vi "Begin.vi"(11 "Image Size":T1=enum."160x120") -> (0 "error out":errorcluster)   [LabVIEW 2011]
doc: "Called before other user functions, this VI is expected to open initial I/O refnums, load in file data, and do all program initialization. Notice that the <B>error out</B> terminal is simply used for data flow. Wiring it to other structures or subVIs ensures that this VI runs first."
uses:
  <vilib>/Rock Robotics/WPI/Camera/WPI_CameraImageSize.ctl
  <vilib>/Rock Robotics/WPI/Solenoid/WPI_SolenoidChannel.ctl
  <vilib>/Rock Robotics/SystemInterfaces/Typedef/FPGA_TypedefSolenoidModule.ctl
  <vilib>/Rock Robotics/SystemInterfaces/DIO/FPGA_DIOChannel.ctl
  <vilib>/Rock Robotics/SystemInterfaces/Typedef/FPGA_TypedefDigitalModule.ctl
  <vilib>/Rock Robotics/WPI/Solenoid/WPI_SolenoidValue.ctl
  <vilib>/Rock Robotics/WPI/CAN/Jaguar/SubVIs/WPI_CANJaguar_BrakeCoastMode.ctl
  <vilib>/Rock Robotics/WPI/CAN/Jaguar/SubVIs/WPI_CANJaguar_ControlMode.ctl
  <vilib>/Rock Robotics/WPI/Encoder/WPI_EncoderType.ctl
  <vilib>/Rock Robotics/WPI/Joystick/WPI_JoystickDeviceEnum.ctl
  <vilib>/Rock Robotics/SystemInterfaces/DIO/FPGA_DIOPWMChannel.ctl
  <vilib>/Rock Robotics/WPI/Relay/WPI_RelayDirection.ctl
  <vilib>/Rock Robotics/SystemInterfaces/DIO/FPGA_DIORelayChannel.ctl
  <vilib>/Rock Robotics/WPI/Solenoid/WPI_SolenoidOpenDouble.vi
  <vilib>/Rock Robotics/WPI/Counter/WPI_CounterDigitalInputToDigitalSource.vi
  <vilib>/Rock Robotics/WPI/Counter/WPI_CounterOpen Semi Period Mode.vi
  <vilib>/Rock Robotics/WPI/Solenoid/WPI_SolenoidSetEnum.vi
  <vilib>/Rock Robotics/WPI/MotorControl/WPI_MotorControlOpenCANJaguar.vi
  <vilib>/Rock Robotics/WPI/RobotDrive/WPI_RobotDriveOpen4MotorWithJaguar.vi
  <vilib>/Rock Robotics/WPI/Camera/WPI_CameraWhite Balance Values.ctl
  <vilib>/Rock Robotics/WPI/Camera/WPI_CameraExposure Values.ctl
  <vilib>/Rock Robotics/WPI/Camera/WPI_CameraFrameRate.ctl
  <vilib>/Rock Robotics/SystemInterfaces/Typedef/FPGA_TypedefAnalogModuleForGyro.ctl
  <vilib>/Rock Robotics/SystemInterfaces/AI/FPGA_AIGyroChannel.ctl
  <vilib>/Rock Robotics/SystemInterfaces/AI/FPGA_AIChannel.ctl
  <vilib>/Rock Robotics/SystemInterfaces/Typedef/FPGA_TypedefAnalogModule.ctl
  <vilib>/Rock Robotics/WPI/MotorControl/WPI_MotorControlOpen Jaguar.vi
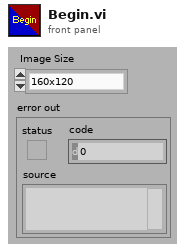
[diagram p1: front panel]
types:
  T1 = typedef "WPI_CameraImageSize.ctl" = enum16{"640x480", "320x240", "160x120"}
  T2 = typedef "FPGA_TypedefDigitalModule.ctl" = enum16{"Digital Module 1", "Digital Module 2"}
  T3 = typedef "FPGA_DIOChannel.ctl" = enum8{"DIO 1", "DIO 2", "DIO 3", "DIO 4", "DIO 5", "DIO 6", "DIO 7", "DIO 8", "DIO 9", "DIO 10", "DIO 11", "DIO 12", "DIO 13", "DIO 14", "Invalid"}
  T4 = typedef "WPI_DigitalInputDevRef.ctl" = cluster{"DevStatus":errorcluster, "DIO Channel":T3, "Digital Module":T2}
  T5 = typedef "WPI_JoystickDeviceEnum.ctl" = enum16{"USB 1", "USB 2", "USB 3", "USB 4", "Kinect 1", "Kinect 2"}
  T6 = typedef "WPI_SolenoidChannel.ctl" = enum8{"Solenoid 1", "Solenoid 2", "Solenoid 3", "Solenoid 4", "Solenoid 5", "Solenoid 6", "Solenoid 7", "Solenoid 8", "Invalid"}
  T7 = typedef "FPGA_TypedefSolenoidModule.ctl" = enum16{"Solenoid Module 1", "Solenoid Module 2"}
  T8 = typedef "FPGA_DIORelayChannel.ctl" = enum8{"Relay 1", "Relay 2", "Relay 3", "Relay 4", "Relay 5", "Relay 6", "Relay 7", "Relay 8", "Invalid"}
  T9 = typedef "WPI_RelayDirection.ctl" = enum16{"Both directions", "Forward only", "Reverse only"}
  T10 = typedef "WPI_EncoderType.ctl" = enum16{"1x", "2x", "4x"}
  T11 = typedef "FPGA_DIOPWMChannel.ctl" = enum8{"PWM 1", "PWM 2", "PWM 3", "PWM 4", "PWM 5", "PWM 6", "PWM 7", "PWM 8", "PWM 9", "PWM 10", "Invalid"}
  T12 = typedef "WPI_JoystickDevRef.ctl" = cluster{"Device":T5}
  T13 = typedef "WPI_RobotDriveDevRef.ctl" = cluster{"DevStatus":errorcluster, "Motors[]":T14[], "Square Inputs":bool, "Max Output":dbl, "Isochronous":bool}
  T14 = typedef "WPI_MotorControlDeviceRef.ctl" = cluster{"DeviceStatus":errorcluster, "Type":enum16{"PWM", "CAN"}, "PWM":cluster{"Digital Module":T2, "PWM Channel":T11, "DeadBand":T15}, "CAN":cluster{"Device Number":u8, "Control Mode":T16, "Semaphore":T17, "Max Vout":dbl}, "Invert":bool, "TransformRef":T18, "InvTransformRef":T18}
  T15 = typedef "WPI_PWMDeadband.ctl" = cluster{"Name":string, "maxPositivePwm":i32, "minPositivePwm":i32, "centerPwm":i32, "maxNegativePwm":i32, "minNegativePwm":i32, "angularRange":u16}
  T16 = typedef "WPI_CANJaguar_ControlMode.ctl" = enum8{"Percent VBus", "Current", "Speed", "Position", "Voltage"}
  T17 = typedef "Semaphore RefNum" = refnum<k1>
  T18 = typedef "WPI_PWMTransform_ConPane.ctl" = refnum<vi>
  T19 = typedef "WPI_SolenoidDevRef.ctl" = cluster{"DevStatus":errorcluster, "Solenoid Module":T7, "Forward Solenoid Channel":T6, "Reverse Solenoid Channel":T6}
  T20 = typedef "WPI_RelayDevRef.ctl" = cluster{"DevStatus":errorcluster, "Relay Channel":T8, "Digital Module":T2, "Relay Direction":T9}
  T21 = typedef "FPGA_CounterEncoderSourceConvertionLVSourceType.ctl" = cluster{"DevStatus":errorcluster, "AnalogTriggerMode?":bool, "DigitalMode":cluster{"Digital Module":T2, "DIO Channel":T22}, "AnalogTriggerMode":cluster{"AnalogTriggerIndex":T23, "OutputType":T24}}
  T22 = typedef "FPGA_DIODigitalSourceChannel.ctl" = enum8{"DIO 1", "DIO 2", "DIO 3", "DIO 4", "DIO 5", "DIO 6", "DIO 7", "DIO 8", "DIO 9", "DIO 10", "DIO 11", "DIO 12", "DIO 13", "DIO 14", "Disabled"}
  T23 = typedef "FPGA_AnalogTriggerIndex.ctl" = enum8{"Trig 0", "Trig 1", "Trig 2", "Trig 3", "Trig 4", "Trig 5", "Trig 6", "Trig 7", "Invalid"}
  T24 = typedef "FPGA_AnalogTriggerOutType.ctl" = enum16{"InWindow", "TriggerState", "Rising", "Falling"}
  T25 = typedef "WPI_EncoderDevRef.ctl" = cluster{"DevStatus":errorcluster, "EncoderIndex":T26, "CounterIndex":T27, "DistancePerCount":dbl, "Decoding Type":T10}
  T26 = typedef "FPGA_EncoderIdx.ctl" = enum8{"Enc 0", "Enc 1", "Enc 2", "Enc 3", "Invalid"}
  T27 = typedef "FPGA_CounterCtrSystemIndex.ctl" = enum8{"Ctr 0", "Ctr 1", "Ctr 2", "Ctr 3", "Ctr 4", "Ctr 5", "Ctr 6", "Ctr 7", "Invalid"}
  T28 = typedef "FPGA_AIChannel.ctl" = enum8{"AI 1", "AI 2", "AI 3", "AI 4", "AI 5", "AI 6", "AI 7", "AI 8", "Invalid"}
  T29 = typedef "FPGA_TypedefAnalogModule.ctl" = enum16{"Analog Module 1", "Analog Module 2"}
  T30 = typedef "FPGA_AIGyroChannel.ctl" = enum8{"AI 1", "AI 2", "Invalid"}
  T31 = typedef "FPGA_TypedefAnalogModuleForGyro.ctl" = enum16{"Analog Module 1"}
  T32 = typedef "WPI_AnalogChannelDevRef.ctl" = cluster{"DevStatus":errorcluster, "Analog Module":T29, "Analog Channel":T28}
  T33 = typedef "WPI_GyroDevRef.ctl" = cluster{"DevStatus":errorcluster, "Analog Module":T29, "Analog Channel":T28, "Offset":dbl, "Gain (VoltsPerDegree/Second)":dbl}
  T34 = cluster{"Channel 1":enum16{"Input (floating)", "Input (pulled high)", "Input (pulled low)", "Output", "PWM"}, "Channel 2":enum16{"Input (floating)", "Input (pulled high)", "Input (pulled low)", "Output", "PWM"}, "Channel 3":enum16{"Input (floating)", "Input (pulled high)", "Input (pulled low)", "Output", "PWM"}, "Channel 4":enum16{"Input (floating)", "Input (pulled high)", "Input (pulled low)", "Output", "PWM"}, "Channel 5":enum16{"Input (floating)", "Input (pulled high)", "Input (pulled low)", "Output"}, "Channel 6":enum16{"Input (floating)", "Input (pulled high)", "Input (pulled low)", "Output"}, "Channel 7":enum16{"Input (floating)", "Input (pulled high)", "Input (pulled low)", "Output"}, "Channel 8":enum16{"Input (floating)", "Input (pulled high)", "Input (pulled low)", "Output"}, "Channel 9":enum16{"Input (floating)", "Input (pulled high)", "Input (pulled low)", "Output"}, "Channel 10":enum16{"Input (floating)", "Input (pulled high)", "Input (pulled low)", "Output"}, "Channel 11":enum16{"Input (floating)", "Input (pulled high)", "Input (pulled low)", "Output"}, "Channel 12":enum16{"Input (floating)", "Input (pulled high)", "Input (pulled low)", "Output"}, "Channel 13":enum16{"Input (floating)", "Input (pulled high)", "Input (pulled low)", "Output"}, "Channel 14":enum16{"Input (floating)", "Input (pulled high)", "Input (pulled low)", "Output"}, "Channel 15":enum16{"Input (floating)", "Input (pulled high)", "Input (pulled low)", "Output", "Analog Comparator"}, "Channel 16":enum16{"Input (floating)", "Input (pulled high)", "Input (pulled low)", "Output", "Analog Comparator"}}
  T35 = cluster{"Period 1(sec)":dbl, "Period 2(sec)":dbl}
  T36 = cluster{"Index Enable 1":bool, "Index Enable 2":bool}
  T37 = typedef "WPI_CameraFrameRate.ctl" = u32
  T38 = typedef "WPI_CameraExposure Values.ctl" = enum16{"Auto", "Flicker-free 50 Hz", "Flicker-free 60 Hz", "Hold current"}
  T39 = typedef "WPI_CameraWhite Balance Values.ctl" = enum16{"Auto", "Fixed indoor", "Fixed outdoor 1", "Fixed outdoor 2", "Fixed fluorescent 1", "Fixed fluorescent 2", "Hold current"}
  T40 = typedef "WPI_CameraDevRef.ctl" = cluster{"Camera Address":string, "CameraStatus":errorcluster, "Acquire Image Notifier":refnum<notifier>}
  T41 = typedef "WPI_SolenoidValue.ctl" = enum16{"Off", "On", "Forward", "Reverse"}
  T42 = typedef "WPI_CounterDevRef.ctl" = cluster{"DevStatus":errorcluster, "CntIndex":T27}
  T43 = typedef "WPI_CANJaguar_BrakeCoastMode.ctl" = enum8{"Jumper", "Brake", "Coast"}
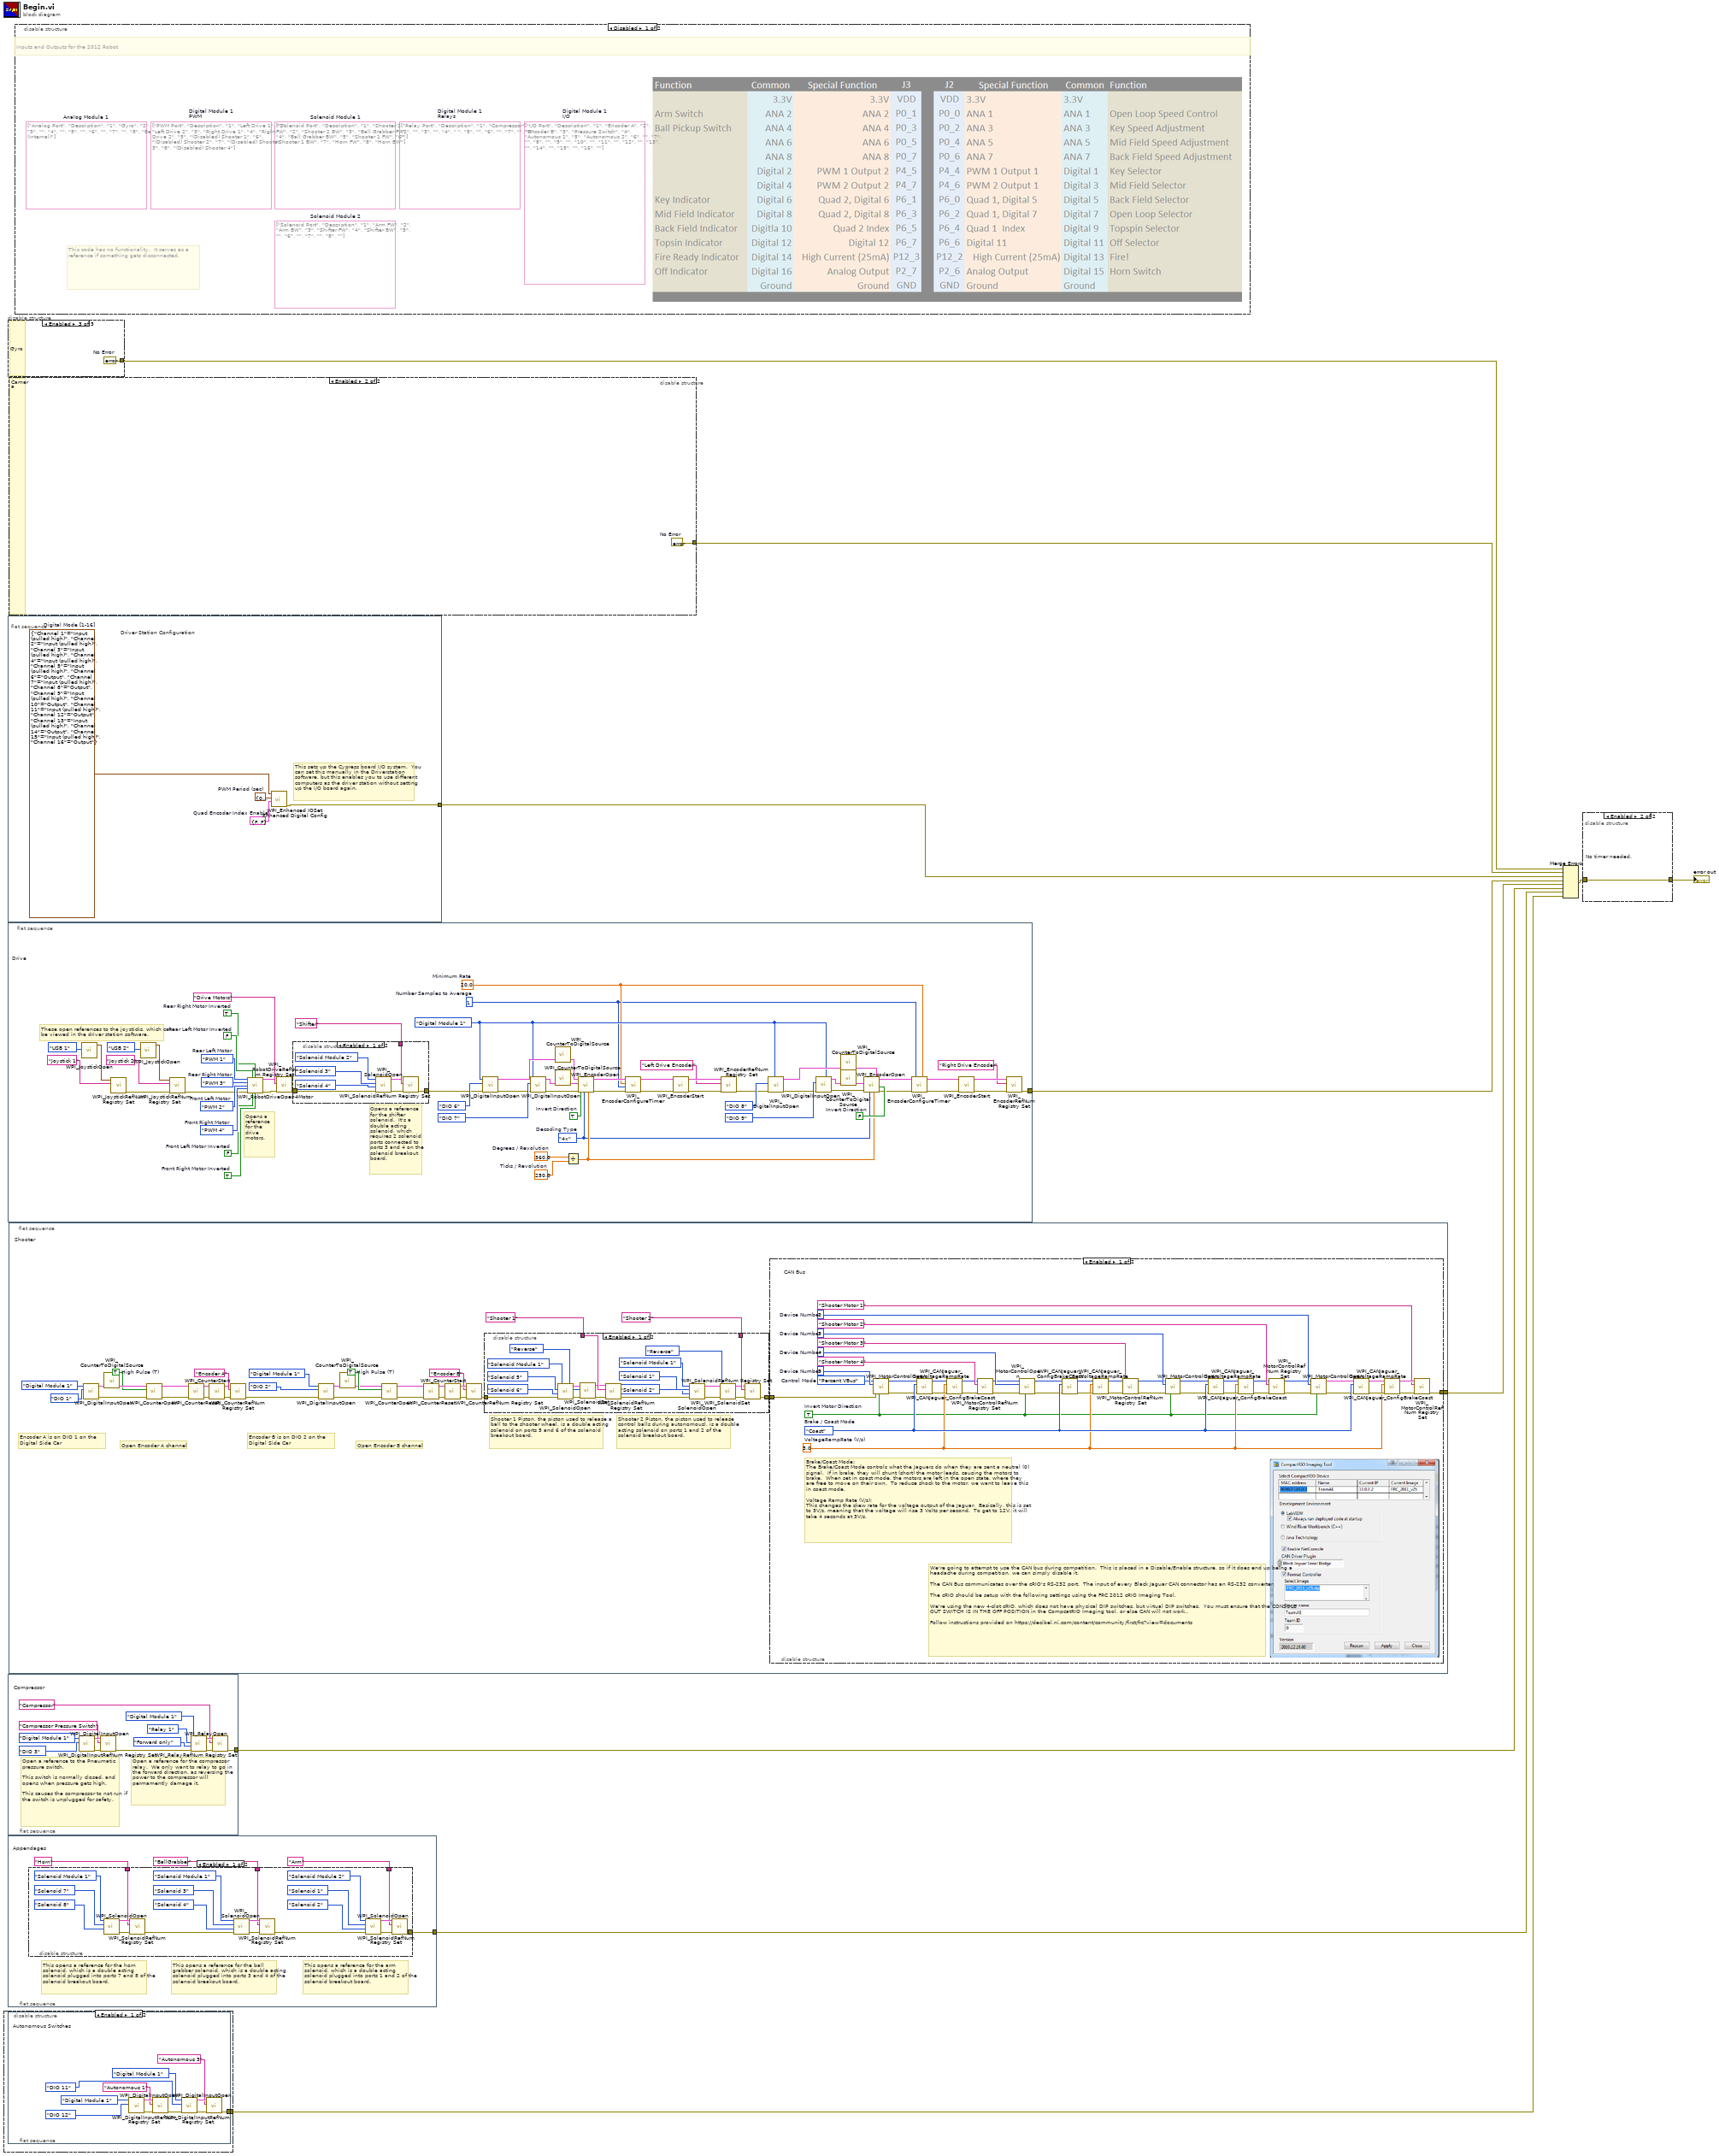
[diagram p0: block diagram]
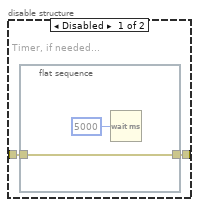
[diagram p4: hidden frame]
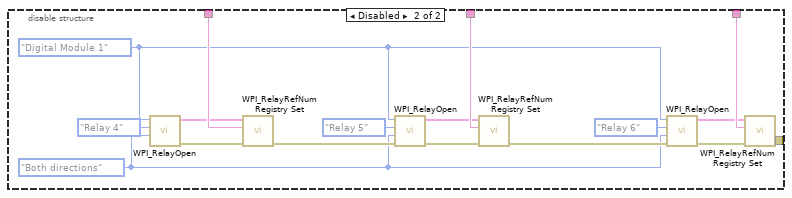
[diagram p5: hidden frame]
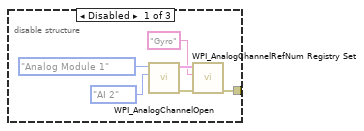
[diagram p6: hidden frame]
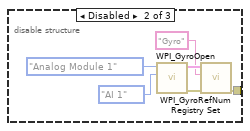
[diagram p7: hidden frame]
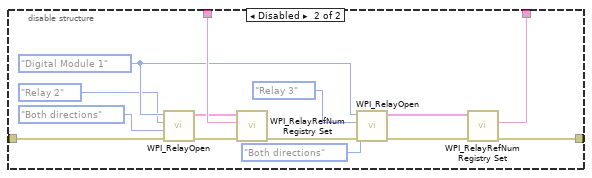
[diagram p8: hidden frame]
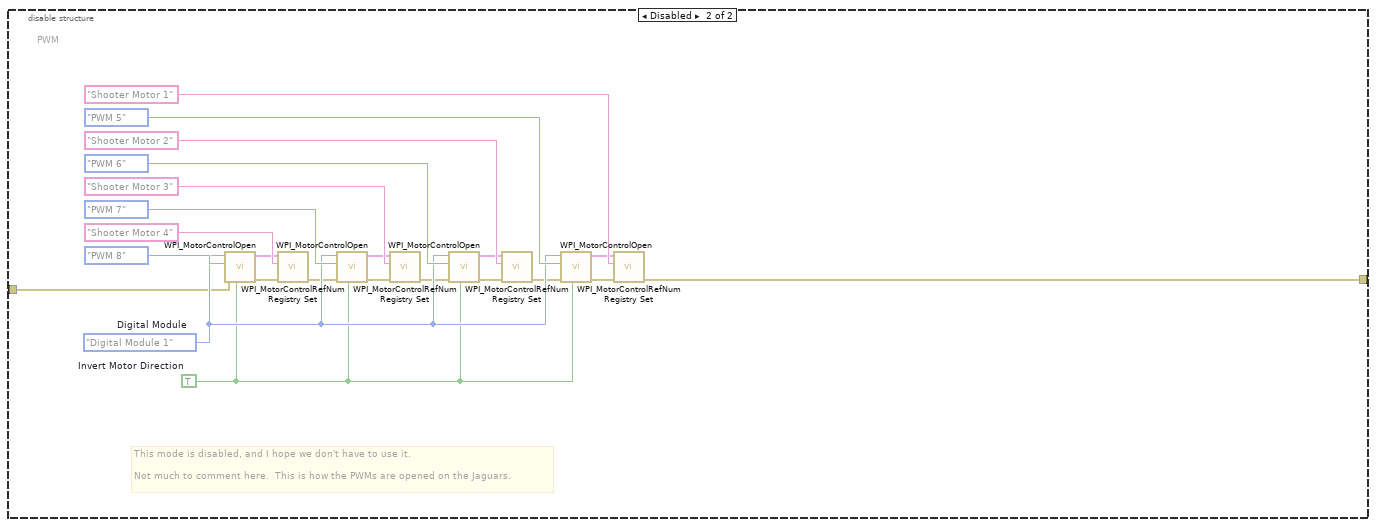
[diagram p9: hidden frame]
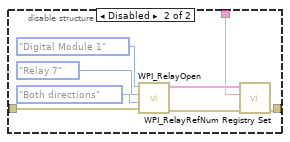
[diagram p10: hidden frame]
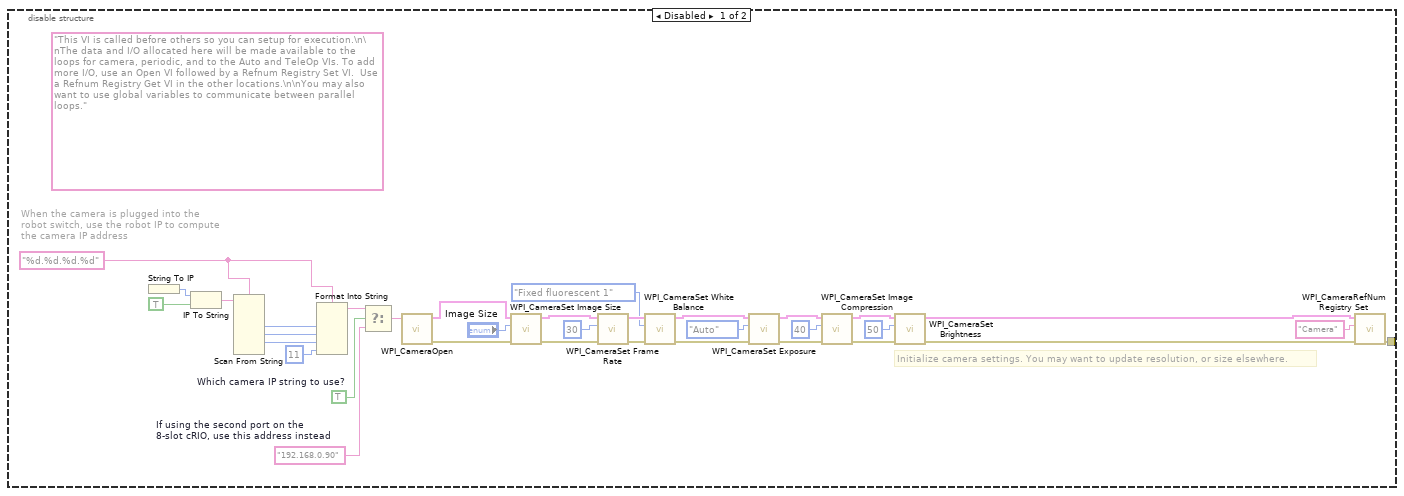
[diagram p11: hidden frame]
diagram:
  n1 = disable-structure shown="Enabled" {
    disable-tunnel: [w11 _] -> w1
    frame Enabled {
      n2 = flat-sequence {
        tunnel: [w12] -> w11
        frame #0 {
          # "Autonomous Switches"
          n3 = call <vilib>:"WPI_DigitalInputOpen.vi"("DIO Channel"=FPGA_DIOChannel."DIO 12", "Digital Module (Module 1)"=FPGA_TypedefDigitalModule."Digital Module 1") -> ("error out"=w19:errorcluster, "DigitalInputDevRef"=w20:T4)  [unwired: 8 in]
          n4 = call <vilib>:"WPI_DigitalInputRefNum Registry Set.vi"("error in (no error)"=w19, "refnum name"="Autonomous 1", "DigitalInputDevRef"=w20) -> ("error out"=w23:errorcluster)  [unwired: 7 in, 1 out]
          n5 = call <vilib>:"WPI_DigitalInputOpen.vi"("error in (no error)"=w23, "DIO Channel"=FPGA_DIOChannel."DIO 11", "Digital Module (Module 1)"=FPGA_TypedefDigitalModule."Digital Module 1") -> ("error out"=w21:errorcluster, "DigitalInputDevRef"=w22:T4)  [unwired: 7 in]
          n6 = call <vilib>:"WPI_DigitalInputRefNum Registry Set.vi"("error in (no error)"=w21, "refnum name"="Autonomous 3", "DigitalInputDevRef"=w22) -> ("error out"=w12:errorcluster)  [unwired: 7 in, 1 out]
        }
      }
    }
    frame Disabled {
    }
  }
  n7 = flat-sequence {
    tunnel: [w35] -> w9
    frame #0 {
      w24 = u8 1  # Number Samples to Average
      w25 = 20.0  # Minimum Rate
      w64 = 250.0  # Ticks / Revolution
      w52 = TRUE  # Invert Direction
      w61 = FALSE  # Invert Direction
      w27 = WPI_EncoderType."4x"  # Decoding Type
      w26 = FPGA_TypedefDigitalModule."Digital Module 1" ("DIO Module")
      w65 = 360.0  # Degrees / Revolution
      w73 = TRUE  # Front Right Motor Inverted
      w74 = FALSE  # Front Left Motor Inverted
      w75 = TRUE  # Rear Right Motor Inverted
      w76 = FALSE  # Rear Left Motor Inverted
      w77 = FPGA_DIOPWMChannel."PWM 4"  # Front Right Motor
      w78 = FPGA_DIOPWMChannel."PWM 2"  # Front Left Motor
      w79 = FPGA_DIOPWMChannel."PWM 3"  # Rear Right Motor
      w80 = FPGA_DIOPWMChannel."PWM 1"  # Rear Left Motor
      # "Opens a reference for the shifter solenoid.  It's a double acting solenoid, which requires 2 solenoid ports connected to ports 3 and 4 on the solenoid breakout board."
      # "Opens a reference for the drive motors."
      # "These open references to the joysticks, which can be viewed in the driver station software."
      # "Drive"
      n8 = call <vilib>:"WPI_JoystickOpen.vi"("JoystickDevice"=WPI_JoystickDeviceEnum."USB 1") -> ("JoystickDevRef"=w85:T12)  [unwired: 10 out]
      n9 = call <vilib>:"WPI_JoystickRefNum Registry Set.vi"("refnum name"="Joystick 1", "JoystickDevRef"=w85) -> ("error out"=w66:errorcluster)  [unwired: 1 in, 8 out]
      n10 = call <vilib>:"WPI_JoystickOpen.vi"("JoystickDevice"=WPI_JoystickDeviceEnum."USB 2") -> ("JoystickDevRef"=w71:T12)  [unwired: 10 out]
      n11 = call <vilib>:"WPI_JoystickRefNum Registry Set.vi"("error in (no error)"=w66, "refnum name"="Joystick 2", "JoystickDevRef"=w71) -> ("error out"=w67:errorcluster)  [unwired: 8 out]
      n12 = call-poly <vilib>:"WPI_RobotDriveOpen4Motor.vi"("Rear Left Motor"=w80, "Rear Left Motor Inverted"=w76, "Rear Right Motor Inverted"=w75, "Rear Right Motor"=w79, "Front Left Motor"=w78, "Front Right Motor"=w77, "error in (no error)"=w67, "Front Left Motor Inverted"=w74, "Front Right Motor Inverted"=w73) -> ("RobotDriveDevRef"=w82:T13, "error out"=w81:errorcluster)  [unwired: 5 in]
      n13 = call <vilib>:"WPI_RobotDriveRefNum Registry Set.vi"("error in (no error)"=w81, "refnum name"="Drive Motors", "RobotDriveDevRef"=w82) -> ("error out"=w68:errorcluster)  [unwired: 8 out]
      n14 = disable-structure shown="Enabled" {
        disable-tunnel: "Shifter" ("refnum name") -> [w93 w98]
        disable-tunnel: w68 -> [w88 w102]
        disable-tunnel: [w87 w100] -> w34
        frame Enabled {
          n15 = call-poly <vilib>:"WPI_SolenoidOpen.vi"("error in (no error)"=w88, "Reverse Solenoid Channel"=WPI_SolenoidChannel."Solenoid 4", "Forward Solenoid Channel"=WPI_SolenoidChannel."Solenoid 3", "Solenoid Module (Module 1)"=FPGA_TypedefSolenoidModule."Solenoid Module 2") -> ("error out"=w91:errorcluster, "SolenoidDevRef"=w90:T19)  [unwired: 6 in]
          n16 = call <vilib>:"WPI_SolenoidRefNum Registry Set.vi"("error in (no error)"=w91, "refnum name"=w93, "SolenoidDevRef"=w90) -> ("error out"=w87:errorcluster)  [unwired: 7 in, 1 out]
        }
        frame Disabled {
          n17 = call <vilib>:"WPI_RelayOpen.vi"("error in (no error)"=w102, "Relay Direction"=WPI_RelayDirection."Both directions", "Relay Channel"=FPGA_DIORelayChannel."Relay 7", "Digital Module (Module 1)"=FPGA_TypedefDigitalModule."Digital Module 1") -> ("error out"=w101:errorcluster, "RelayDevRef"=w99:T20)  [unwired: 6 in]
          n18 = call <vilib>:"WPI_RelayRefNum Registry Set.vi"("error in (no error)"=w101, "refnum name"=w98, "RelayDevRef"=w99) -> ("error out"=w100:errorcluster)  [unwired: 7 in, 1 out]
        }
      }
      n19 = call <vilib>:"WPI_DigitalInputOpen.vi"("error in (no error)"=w34, "DIO Channel"=FPGA_DIOChannel."DIO 6", "Digital Module (Module 1)"=w26) -> ("error out"=w33:errorcluster, "DigitalInputDevRef"=w50:T4)  [unwired: 7 out]
      n20 = call <vilib>:"WPI_DigitalInputOpen.vi"("error in (no error)"=w33, "DIO Channel"=FPGA_DIOChannel."DIO 7", "Digital Module (Module 1)"=w26) -> ("error out"=w32:errorcluster, "DigitalInputDevRef"=w49:T4)  [unwired: 7 out]
      n21 = call-poly <vilib>:"WPI_CounterToDigitalSource.vi"("DigitalInputDevRef"=w50) -> ("Digital Source"=w51:T21)  [unwired: 6 out]
      n22 = call-poly <vilib>:"WPI_CounterToDigitalSource.vi"("DigitalInputDevRef"=w49) -> ("Digital Source"=w48:T21)  [unwired: 6 out]
      n23 = Divide(x=w65, y=w64) -> (x/y=w28:dbl)
      n24 = call <vilib>:"WPI_EncoderOpen.vi"("DistancePerCount"=w28, "Decoding Type"=w27, "error in (no error)"=w32, "Invert Direction (False)"=w52, "BSource"=w48, "ASource"=w51) -> ("error out"=w47:errorcluster, "EncoderDevRef"=w46:T25)  [unwired: 2 in, 2 out]
      n25 = call <vilib>:"WPI_EncoderConfigureTimer.vi"("error in (no error)"=w47, "Number Samples to Average"=w24, "Minimum Rate"=w25, "EncoderDevRef"=w46) -> ("error out"=w42:errorcluster, "EncoderDevRef"=w45:T25)  [unwired: 6 out]
      n26 = call <vilib>:"WPI_EncoderStart.vi"("error in (no error)"=w42, "EncoderDevRef"=w45) -> ("error out"=w41:errorcluster, "EncoderDevRef"=w40:T25)  [unwired: 8 out]
      n27 = call <vilib>:"WPI_EncoderRefNum Registry Set.vi"("error in (no error)"=w41, "refnum name"="Left Drive Encoder", "EncoderDevRef"=w40) -> ("error out"=w31:errorcluster)  [unwired: 7 in, 1 out]
      n28 = call <vilib>:"WPI_DigitalInputOpen.vi"("error in (no error)"=w31, "DIO Channel"=FPGA_DIOChannel."DIO 8" ("Encoder A Channel"), "Digital Module (Module 1)"=w26) -> ("error out"=w30:errorcluster, "DigitalInputDevRef"=w58:T4)  [unwired: 7 out]
      n29 = call <vilib>:"WPI_DigitalInputOpen.vi"("error in (no error)"=w30, "DIO Channel"=FPGA_DIOChannel."DIO 9" ("Encoder B Channel"), "Digital Module (Module 1)"=w26) -> ("error out"=w29:errorcluster, "DigitalInputDevRef"=w59:T4)  [unwired: 7 out]
      n30 = call-poly <vilib>:"WPI_CounterToDigitalSource.vi"("DigitalInputDevRef"=w58) -> ("Digital Source"=w57:T21)  [unwired: 6 out]
      n31 = call-poly <vilib>:"WPI_CounterToDigitalSource.vi"("DigitalInputDevRef"=w59) -> ("Digital Source"=w60:T21)  [unwired: 6 out]
      n32 = call <vilib>:"WPI_EncoderOpen.vi"("DistancePerCount"=w28, "Decoding Type"=w27, "error in (no error)"=w29, "Invert Direction (False)"=w61, "BSource"=w60, "ASource"=w57) -> ("error out"=w44:errorcluster, "EncoderDevRef"=w55:T25)  [unwired: 2 in, 2 out]
      n33 = call <vilib>:"WPI_EncoderConfigureTimer.vi"("error in (no error)"=w44, "Number Samples to Average"=w24, "Minimum Rate"=w25, "EncoderDevRef"=w55) -> ("error out"=w43:errorcluster, "EncoderDevRef"=w56:T25)  [unwired: 6 out]
      n34 = call <vilib>:"WPI_EncoderStart.vi"("error in (no error)"=w43, "EncoderDevRef"=w56) -> ("error out"=w39:errorcluster, "EncoderDevRef"=w38:T25)  [unwired: 8 out]
      n35 = call <vilib>:"WPI_EncoderRefNum Registry Set.vi"("error in (no error)"=w39, "refnum name"="Right Drive Encoder", "EncoderDevRef"=w38) -> ("error out"=w35:errorcluster)  [unwired: 7 in, 1 out]
    }
  }
  n36 = disable-structure shown="Enabled" {
    disable-tunnel: [w103 w109 w115] -> w2
    frame Disabled {
      n37 = call <vilib>:"WPI_AnalogChannelOpen.vi"("Analog Channel"=FPGA_AIChannel."AI 2", "Analog Module (Module 1)"=FPGA_TypedefAnalogModule."Analog Module 1") -> ("error out"=w104:errorcluster, "AIDeviceRef"=w108:T32)  [unwired: 8 in]
      n38 = call <vilib>:"WPI_AnalogChannelRefNum Registry Set.vi"("error in (no error)"=w104, "refnum name"="Gyro", "AIDeviceRef"=w108) -> ("error out"=w103:errorcluster)  [unwired: 7 in, 1 out]
    }
    frame Disabled {
      n39 = call <vilib>:"WPI_GyroOpen.vi"("Analog Channel"=FPGA_AIGyroChannel."AI 1", "Analog Module (Module 1)"=FPGA_TypedefAnalogModuleForGyro."Analog Module 1") -> ("error out"=w114:errorcluster, "GyroDevRef"=w113:T33)  [unwired: 7 in, 1 out]
      n40 = call <vilib>:"WPI_GyroRefNum Registry Set.vi"("error in (no error)"=w114, "refnum name"="Gyro", "GyroDevRef"=w113) -> ("error out"=w109:errorcluster)  [unwired: 7 in, 1 out]
    }
    frame Enabled {
      w115 = errorcluster {"status"=FALSE, "code"=0, "source"=""}  # No Error
      # "Gyro"
    }
  }
  n41 = flat-sequence {
    tunnel: [w116] -> w10
    frame #0 {
      w117 = T34 {"Channel 1"=enum."Input (pulled high)", "Channel 2"=enum."Input (pulled high)", "Channel 3"=enum."Input (pulled high)", "Channel 4"=enum."Input (pulled high)", "Channel 5"=enum."Input (pulled high)", "Channel 6"=enum."Output", "Channel 7"=enum."Input (pulled high)", "Channel 8"=enum."Output", "Channel 9"=enum."Input (pulled high)", "Channel 10"=enum."Output", "Channel 11"=enum."Input (pulled high)", "Channel 12"=enum."Output", "Channel 13"=enum."Input (pulled high)", "Channel 14"=enum."Output", "Channel 15"=enum."Input (pulled high)", "Channel 16"=enum."Output"}  # Digital Mode [1-16]
      w118 = T35 {"Period 1(sec)"=0.0, "Period 2(sec)"=0.0}  # PWM Period (sec)
      w119 = T36 {"Index Enable 1"=FALSE, "Index Enable 2"=FALSE}  # Quad Encoder Index Enable
      # "This sets up the Cypress board I/O system.  You can set this manually in the Driverstation software, but this enables you to use different computers as the driver station without setting up the I/O board again."
      # "Driver Station Configuration"
      n42 = call <vilib>:"WPI_Enhanced IOSet Enhanced Digital Config.vi"("Quad Encoder Index Enable"=w119, "PWM Period (sec)"=w118, "Digital Mode [1-16]"=w117) -> ("error out"=w116:errorcluster)  [unwired: 8 in]
    }
  }
  n43 = flat-sequence {
    tunnel: [w120] -> w7
    frame #0 {
      # "Open a reference for the compressor relay.  We only want to relay to go in the forward direction, as reversing the power to the compressor will permamently damage it."
      # "Open a reference to the Pneumatic pressure switch.\n\nThis switch is normally closed, and opens when pressure gets high.\n\nThis causes the compressor to not run if the switch is unplugged for safety."
      # "Compressor"
      n44 = call <vilib>:"WPI_DigitalInputOpen.vi"("DIO Channel"=FPGA_DIOChannel."DIO 3", "Digital Module (Module 1)"=FPGA_TypedefDigitalModule."Digital Module 1") -> ("error out"=w125:errorcluster, "DigitalInputDevRef"=w126:T4)  [unwired: 8 in]
      n45 = call <vilib>:"WPI_DigitalInputRefNum Registry Set.vi"("error in (no error)"=w125, "refnum name"="Compressor Pressure Switch", "DigitalInputDevRef"=w126) -> ("error out"=w121:errorcluster)  [unwired: 7 in, 1 out]
      n46 = call <vilib>:"WPI_RelayOpen.vi"("error in (no error)"=w121, "Relay Direction"=WPI_RelayDirection."Forward only", "Relay Channel"=FPGA_DIORelayChannel."Relay 1", "Digital Module (Module 1)"=FPGA_TypedefDigitalModule."Digital Module 1") -> ("error out"=w131:errorcluster, "RelayDevRef"=w132:T20)  [unwired: 6 in]
      n47 = call <vilib>:"WPI_RelayRefNum Registry Set.vi"("error in (no error)"=w131, "refnum name"="Compressor", "RelayDevRef"=w132) -> ("error out"=w120:errorcluster)  [unwired: 7 in, 1 out]
    }
  }
  n48 = flat-sequence {
    tunnel: [w133] -> w6
    frame #0 {
      # "This opens a reference for the arm solenoid, which is a double acting solenoid plugged into ports 1 and 2 of the solenoid breakout board."
      # "This opens a reference for the ball grabber solenoid, which is a double acting solenoid plugged into ports 3 and 4 of the solenoid breakout board."
      # "This opens a reference for the horn solenoid, which is a double acting solenoid plugged into ports 7 and 8 of the solenoid breakout board."
      # "Appendages"
      n49 = disable-structure shown="Enabled" {
        disable-tunnel: "BallGrabber" ("refnum name") -> [w148 w167]
        disable-tunnel: "Horn" ("refnum name") -> [w147 w168]
        disable-tunnel: "Arm" ("refnum name") -> [w146 w166]
        disable-tunnel: [w137 w174] -> w133
        frame Enabled {
          n50 = call-poly <vilib>:"WPI_SolenoidOpen.vi"("Reverse Solenoid Channel"=WPI_SolenoidChannel."Solenoid 8", "Forward Solenoid Channel"=WPI_SolenoidChannel."Solenoid 7", "Solenoid Module (Module 1)"=FPGA_TypedefSolenoidModule."Solenoid Module 1") -> ("error out"=w154:errorcluster, "SolenoidDevRef"=w155:T19)  [unwired: 7 in]
          n51 = call <vilib>:"WPI_SolenoidRefNum Registry Set.vi"("error in (no error)"=w154, "refnum name"=w147, "SolenoidDevRef"=w155) -> ("error out"=w139:errorcluster)  [unwired: 7 in, 1 out]
          n52 = call-poly <vilib>:"WPI_SolenoidOpen.vi"("error in (no error)"=w139, "Reverse Solenoid Channel"=WPI_SolenoidChannel."Solenoid 4", "Forward Solenoid Channel"=WPI_SolenoidChannel."Solenoid 3", "Solenoid Module (Module 1)"=FPGA_TypedefSolenoidModule."Solenoid Module 1") -> ("error out"=w157:errorcluster, "SolenoidDevRef"=w156:T19)  [unwired: 6 in]
          n53 = call <vilib>:"WPI_SolenoidRefNum Registry Set.vi"("error in (no error)"=w157, "refnum name"=w148, "SolenoidDevRef"=w156) -> ("error out"=w138:errorcluster)  [unwired: 7 in, 1 out]
          n54 = call-poly <vilib>:"WPI_SolenoidOpen.vi"("error in (no error)"=w138, "Reverse Solenoid Channel"=WPI_SolenoidChannel."Solenoid 2", "Forward Solenoid Channel"=WPI_SolenoidChannel."Solenoid 1", "Solenoid Module (Module 1)"=FPGA_TypedefSolenoidModule."Solenoid Module 2") -> ("error out"=w152:errorcluster, "SolenoidDevRef"=w153:T19)  [unwired: 6 in]
          n55 = call <vilib>:"WPI_SolenoidRefNum Registry Set.vi"("error in (no error)"=w152, "refnum name"=w146, "SolenoidDevRef"=w153) -> ("error out"=w137:errorcluster)  [unwired: 7 in, 1 out]
        }
        frame Disabled {
          w161 = WPI_RelayDirection."Both directions" ("Relay Direction")
          w162 = FPGA_TypedefDigitalModule."Digital Module 1" ("Digital Module (Module 1)")
          n56 = call <vilib>:"WPI_RelayOpen.vi"("Relay Direction"=w161, "Relay Channel"=FPGA_DIORelayChannel."Relay 4", "Digital Module (Module 1)"=w162) -> ("error out"=w169:errorcluster, "RelayDevRef"=w163:T20)  [unwired: 7 in]
          n57 = call <vilib>:"WPI_RelayRefNum Registry Set.vi"("error in (no error)"=w169, "refnum name"=w168, "RelayDevRef"=w163) -> ("error out"=w170:errorcluster)  [unwired: 7 in, 1 out]
          n58 = call <vilib>:"WPI_RelayOpen.vi"("error in (no error)"=w170, "Relay Direction"=w161, "Relay Channel"=FPGA_DIORelayChannel."Relay 5", "Digital Module (Module 1)"=w162) -> ("error out"=w171:errorcluster, "RelayDevRef"=w164:T20)  [unwired: 6 in]
          n59 = call <vilib>:"WPI_RelayRefNum Registry Set.vi"("error in (no error)"=w171, "refnum name"=w167, "RelayDevRef"=w164) -> ("error out"=w172:errorcluster)  [unwired: 7 in, 1 out]
          n60 = call <vilib>:"WPI_RelayOpen.vi"("error in (no error)"=w172, "Relay Direction"=w161, "Relay Channel"=FPGA_DIORelayChannel."Relay 6", "Digital Module (Module 1)"=w162) -> ("error out"=w173:errorcluster, "RelayDevRef"=w165:T20)  [unwired: 6 in]
          n61 = call <vilib>:"WPI_RelayRefNum Registry Set.vi"("error in (no error)"=w173, "refnum name"=w166, "RelayDevRef"=w165) -> ("error out"=w174:errorcluster)  [unwired: 7 in, 1 out]
        }
      }
    }
  }
  n62 = disable-structure shown="Enabled" {
    disable-tunnel: [w175 w209] -> w3
    frame Disabled {
      w176 = TRUE  # Which camera IP string to use?
      w180 = "%d.%d.%d.%d" ("format string")
      (unwired) "This VI is called before others so you can setup for execution.\n\nThe data and I/O allocated here will be made available to the loops for camera, periodic, and to the Auto and TeleOp VIs. To add more I/O, use an Open VI followed by a Refnum Registry Set VI.  Use a Refnum Registry Get VI in the other locations.\n\nYou may also want to use global variables to communicate between parallel loops."
      w177 = "192.168.0.90"  # If using the second port on the 8-slot cRIO, use this address instead
      # "When the camera is plugged into the\nrobot switch, use the robot IP to compute\nthe camera IP address"
      # "Initialize camera settings. You may want to update resolution, or size elsewhere."
      n63 = String To IP() -> (0:w187:u32)  [unwired: 1 in]
      n64 = IP To String(1:TRUE ("dot notation? (F)"), 2:w187) -> (0:w185:string)
      n65 = Scan From String(format string=w180, input string=w185) -> (output 1=w184:i32, output 2=w183:i32, output 3=w182:i32)  [unwired: 7 in, 3 out]
      n66 = Format Into String(format string=w180, w184, w183, w182, 11 ("Compression")) -> (resulting string=w178:string)  [unwired: 2 in, 1 out]
      n67 = Select(t=w178, s=w176, f=w177) -> (s? t:f=w179:string)
      n68 = call <vilib>:"WPI_CameraOpen.vi"("Camera Address"=w179) -> ("error out"=w199:errorcluster, "CameraDevRef"=w200:T40)  [unwired: 1 in, 8 out]
      n69 = call <vilib>:"WPI_CameraSet Image Size.vi"("error in (no error)"=w199, "Image Size"="Image Size", "CameraDevRef"=w200) -> ("error out"=w198:errorcluster, "CameraDevRef Out"=w201:T40)  [unwired: 7 out]
      n70 = call <vilib>:"WPI_CameraSet Frame Rate.vi"("error in (no error)"=w198, "Frame Rate (fps)"=T37 30, "CameraDevRef"=w201) -> ("error out"=w197:errorcluster, "CameraDevRef Out"=w203:T40)  [unwired: 7 out]
      n71 = call <vilib>:"WPI_CameraSet White Balance.vi"("error in (no error)"=w197, "White Balance"=WPI_CameraWhite_Balance_Values."Fixed fluorescent 1", "CameraDevRef"=w203) -> ("error out"=w196:errorcluster, "CameraDevRef Out"=w202:T40)  [unwired: 7 out]
      n72 = call <vilib>:"WPI_CameraSet Exposure.vi"("error in (no error)"=w196, "Exposure"=WPI_CameraExposure_Values."Auto", "CameraDevRef"=w202) -> ("error out"=w195:errorcluster, "CameraDevRef Out"=w205:T40)  [unwired: 7 out]
      n73 = call <vilib>:"WPI_CameraSet Image Compression.vi"("error in (no error)"=w195, "Compression"=40, "CameraDevRef"=w205) -> ("error out"=w194:errorcluster, "CameraDevRef Out"=w204:T40)  [unwired: 7 out]
      n74 = call <vilib>:"WPI_CameraSet Brightness.vi"("error in (no error)"=w194, "Brightness"=50, "CameraDevRef"=w204) -> ("error out"=w192:errorcluster, "CameraDevRef Out"=w193:T40)  [unwired: 7 out]
      n75 = call <vilib>:"WPI_CameraRefNum Registry Set.vi"("error in (no error)"=w192, "refnum name"="Camera", "CameraDevRef"=w193) -> ("error out"=w175:errorcluster)  [unwired: 8 out]
    }
    frame Enabled {
      w209 = errorcluster {"status"=FALSE, "code"=0, "source"=""}  # No Error
      # "Camera"
    }
  }
  n76 = flat-sequence {
    tunnel: [w212] -> w8
    frame #0 {
      w226 = TRUE  # High Pulse (T)
      w231 = TRUE  # High Pulse (T)
      # "Shooter 2 Piston, the piston used to release control balls during autonomousl, is a double acting solenoid on ports 1 and 2 of the solenoid breakout board."
      # "Shooter 1 Piston, the piston used to release a ball to the shooter wheel, is a double acting solenoid on ports 5 and 6 of the solenoid breakout board."
      # "Encoder A is on DIO 1 on the Digital Side Car"
      # "Encoder B is on DIO 2 on the Digital Side Car"
      # "Open Encoder B channel"
      # "Open Encoder A channel"
      # "Shooter"
      n77 = call <vilib>:"WPI_DigitalInputOpen.vi"("DIO Channel"=FPGA_DIOChannel."DIO 1", "Digital Module (Module 1)"=FPGA_TypedefDigitalModule."Digital Module 1") -> ("error out"=w232:errorcluster, "DigitalInputDevRef"=w233:T4)  [unwired: 8 in]
      n78 = call-poly <vilib>:"WPI_CounterToDigitalSource.vi"("DigitalInputDevRef"=w233) -> ("Digital Source"=w241:T21)  [unwired: 6 in]
      n79 = call-poly <vilib>:"WPI_CounterOpen.vi"("error in (no error)"=w232, "High Pulse (T)"=w231, "Source"=w241) -> ("error out"=w237:errorcluster, "CounterDevRef"=w238:T42)  [unwired: 7 in]
      n80 = call <vilib>:"WPI_CounterReset.vi"("error in (no error)"=w237, "CounterDevRef in"=w238) -> ("error out"=w236:errorcluster, "CounterDevRef out"=w239:T42)  [unwired: 8 in]
      n81 = call <vilib>:"WPI_CounterStart.vi"("error in (no error)"=w236, "CounterDevRef in"=w239) -> ("error out"=w234:errorcluster, "CounterDevRef out"=w235:T42)  [unwired: 8 in]
      n82 = call <vilib>:"WPI_CounterRefNum Registry Set.vi"("error in (no error)"=w234, "refnum name"="Encoder A", "CounterDevRef"=w235) -> ("error out"=w215:errorcluster)  [unwired: 7 in, 1 out]
      n83 = call <vilib>:"WPI_DigitalInputOpen.vi"("error in (no error)"=w215, "DIO Channel"=FPGA_DIOChannel."DIO 2", "Digital Module (Module 1)"=FPGA_TypedefDigitalModule."Digital Module 1") -> ("error out"=w225:errorcluster, "DigitalInputDevRef"=w224:T4)  [unwired: 7 in]
      n84 = call-poly <vilib>:"WPI_CounterToDigitalSource.vi"("DigitalInputDevRef"=w224) -> ("Digital Source"=w216:T21)  [unwired: 6 in]
      n85 = call-poly <vilib>:"WPI_CounterOpen.vi"("error in (no error)"=w225, "High Pulse (T)"=w226, "Source"=w216) -> ("error out"=w220:errorcluster, "CounterDevRef"=w219:T42)  [unwired: 7 in]
      n86 = call <vilib>:"WPI_CounterReset.vi"("error in (no error)"=w220, "CounterDevRef in"=w219) -> ("error out"=w221:errorcluster, "CounterDevRef out"=w218:T42)  [unwired: 8 in]
      n87 = call <vilib>:"WPI_CounterStart.vi"("error in (no error)"=w221, "CounterDevRef in"=w218) -> ("error out"=w223:errorcluster, "CounterDevRef out"=w222:T42)  [unwired: 8 in]
      n88 = call <vilib>:"WPI_CounterRefNum Registry Set.vi"("error in (no error)"=w223, "refnum name"="Encoder B", "CounterDevRef"=w222) -> ("error out"=w214:errorcluster)  [unwired: 7 in, 1 out]
      n89 = disable-structure shown="Enabled" {
        disable-tunnel: w214 -> [w256 w274]
        disable-tunnel: [w254 w270] -> w213
        disable-tunnel: "Shooter 2" ("refnum name") -> [w253 w275]
        disable-tunnel: "Shooter 1" ("refnum name") -> [w252 w276]
        frame Enabled {
          n90 = call-poly <vilib>:"WPI_SolenoidOpen.vi"("error in (no error)"=w256, "Reverse Solenoid Channel"=WPI_SolenoidChannel."Solenoid 6", "Forward Solenoid Channel"=WPI_SolenoidChannel."Solenoid 5", "Solenoid Module (Module 1)"=FPGA_TypedefSolenoidModule."Solenoid Module 1") -> ("error out"=w249:errorcluster, "SolenoidDevRef"=w250:T19)  [unwired: 6 in]
          n91 = call-poly <vilib>:"WPI_SolenoidSet.vi"("error in (no error)"=w249, "Value"=WPI_SolenoidValue."Reverse", "SolenoidDevRef"=w250) -> ("error out"=w247:errorcluster, "SolenoidDevRef"=w248:T19)  [unwired: 7 in]
          n92 = call <vilib>:"WPI_SolenoidRefNum Registry Set.vi"("error in (no error)"=w247, "refnum name"=w252, "SolenoidDevRef"=w248) -> ("error out"=w255:errorcluster)  [unwired: 7 in, 1 out]
          n93 = call-poly <vilib>:"WPI_SolenoidOpen.vi"("error in (no error)"=w255, "Reverse Solenoid Channel"=WPI_SolenoidChannel."Solenoid 2", "Forward Solenoid Channel"=WPI_SolenoidChannel."Solenoid 1", "Solenoid Module (Module 1)"=FPGA_TypedefSolenoidModule."Solenoid Module 1") -> ("error out"=w242:errorcluster, "SolenoidDevRef"=w245:T19)  [unwired: 6 in]
          n94 = call-poly <vilib>:"WPI_SolenoidSet.vi"("error in (no error)"=w242, "Value"=WPI_SolenoidValue."Reverse", "SolenoidDevRef"=w245) -> ("error out"=w243:errorcluster, "SolenoidDevRef"=w244:T19)  [unwired: 7 in]
          n95 = call <vilib>:"WPI_SolenoidRefNum Registry Set.vi"("error in (no error)"=w243, "refnum name"=w253, "SolenoidDevRef"=w244) -> ("error out"=w254:errorcluster)  [unwired: 7 in, 1 out]
        }
        frame Disabled {
          w267 = FPGA_TypedefDigitalModule."Digital Module 1" ("Digital Module (Module 1)")
          n96 = call <vilib>:"WPI_RelayOpen.vi"("error in (no error)"=w274, "Relay Direction"=WPI_RelayDirection."Both directions", "Relay Channel"=FPGA_DIORelayChannel."Relay 2", "Digital Module (Module 1)"=w267) -> ("error out"=w273:errorcluster, "RelayDevRef"=w268:T20)  [unwired: 6 in]
          n97 = call <vilib>:"WPI_RelayRefNum Registry Set.vi"("error in (no error)"=w273, "refnum name"=w276, "RelayDevRef"=w268) -> ("error out"=w272:errorcluster)  [unwired: 7 in, 1 out]
          n98 = call <vilib>:"WPI_RelayOpen.vi"("error in (no error)"=w272, "Relay Direction"=WPI_RelayDirection."Both directions", "Relay Channel"=FPGA_DIORelayChannel."Relay 3", "Digital Module (Module 1)"=w267) -> ("error out"=w271:errorcluster, "RelayDevRef"=w269:T20)  [unwired: 6 in]
          n99 = call <vilib>:"WPI_RelayRefNum Registry Set.vi"("error in (no error)"=w271, "refnum name"=w275, "RelayDevRef"=w269) -> ("error out"=w270:errorcluster)  [unwired: 7 in, 1 out]
        }
      }
      n100 = disable-structure shown="Enabled" {
        disable-tunnel: w213 -> [w278 w323]
        disable-tunnel: [w277 w319] -> w212
        frame Enabled {
          w279 = TRUE  # Invert Motor Direction
          w300 = 3.0  # VoltageRampRate (V/s)
          w309 = WPI_CANJaguar_BrakeCoastMode."Coast"  # Brake / Coast Mode
          w310 = WPI_CANJaguar_ControlMode."Percent VBus"  # Control Mode
          w314 = u8 2  # Device Number
          w315 = u8 3  # Device Number
          w316 = u8 4  # Device Number
          w317 = u8 5  # Device Number
          # "Brake/Coast Mode:\nThe Brake/Coast Mode controls what the Jaguars do when they are sent a neutral (0) signal.  If in brake, they will shunt (short) the motor leads, causing the motors to brake.  When set in coast mode, the motors are left in the open state, where they are free to move on their own.  To reduce shock to the motor, we want to leave this in coast mode.\n\nVoltage Ramp Rate (V/s):\nThis changes the skew rate for the voltage output of the Jaguar.  Basically, this is set to 3V/s, meaning that the voltage will rise 3 Volts per second.  To get to 12V, it will take 4 seconds at 3V/s."
          # "We're going to attempt to use the CAN bus during competition.  This is placed in a Disable/Enable structure, so if it does end up being a headache during competition, we can simply disable it.\n\nThe CAN Bus communicates over the cRIO's RS-232 port.  The input of every Black Jaguar CAN connector has an RS-232 converter. \n\nThe cRIO should be setup with the following settings using the FRC 2012 cRIO Imaging Tool.\n\nWe're using the new 4-slot cRIO, which does not have physical DIP switches, but virtual DIP switches.  You must ensure that the CONSOLE OUT SWITCH IS IN THE OFF POSITION in the CompcatRIO Imaging tool, or else CAN will not work..\n\nFollow instructions provided on https://decibel.ni.com/content/community/first/frc?view=documents"
          # "CAN Bus"
          n101 = call-poly <vilib>:"WPI_MotorControlOpen.vi"("Invert"=w279, "error in (no error)"=w278, "Device Number"=w317, "Control Mode"=w310) -> ("error out"=w298:errorcluster, "MotorControlDeviceRef"=w299:T14)  [unwired: 6 in]
          n102 = call <vilib>:"WPI_CANJaguar_ConfigBrakeCoast.vi"("error in (no error)"=w298, "Brake / Coast Mode"=w309, "CAN Jaguar Ref"=w299) -> ("error out"=w307:errorcluster, "CAN Jaguar Ref Out"=w308:T14)  [unwired: 7 in]
          n103 = call <vilib>:"WPI_CANJaguar_SetVoltageRampRate.vi"("error in (no error)"=w307, "VoltageRampRate (V/s)"=w300, "CAN Jaguar Ref"=w308) -> ("error out"=w290:errorcluster, "CAN Jaguar Ref Out"=w291:T14)  [unwired: 7 in]
          n104 = call <vilib>:"WPI_MotorControlRefNum Registry Set.vi"("error in (no error)"=w290, "refnum name"="Shooter Motor 4", "MotorControlDevRef"=w291) -> ("error out"=w283:errorcluster)  [unwired: 7 in, 1 out]
          n105 = call-poly <vilib>:"WPI_MotorControlOpen.vi"("Invert"=w279, "error in (no error)"=w283, "Device Number"=w316, "Control Mode"=w310) -> ("error out"=w296:errorcluster, "MotorControlDeviceRef"=w297:T14)  [unwired: 6 in]
          n106 = call <vilib>:"WPI_CANJaguar_ConfigBrakeCoast.vi"("error in (no error)"=w296, "Brake / Coast Mode"=w309, "CAN Jaguar Ref"=w297) -> ("error out"=w302:errorcluster, "CAN Jaguar Ref Out"=w301:T14)  [unwired: 7 in]
          n107 = call <vilib>:"WPI_CANJaguar_SetVoltageRampRate.vi"("error in (no error)"=w302, "VoltageRampRate (V/s)"=w300, "CAN Jaguar Ref"=w301) -> ("error out"=w288:errorcluster, "CAN Jaguar Ref Out"=w289:T14)  [unwired: 7 in]
          n108 = call <vilib>:"WPI_MotorControlRefNum Registry Set.vi"("error in (no error)"=w288, "refnum name"="Shooter Motor 3", "MotorControlDevRef"=w289) -> ("error out"=w282:errorcluster)  [unwired: 7 in, 1 out]
          n109 = call-poly <vilib>:"WPI_MotorControlOpen.vi"("Invert"=w279, "error in (no error)"=w282, "Device Number"=w315, "Control Mode"=w310) -> ("error out"=w294:errorcluster, "MotorControlDeviceRef"=w295:T14)  [unwired: 6 in]
          n110 = call <vilib>:"WPI_CANJaguar_ConfigBrakeCoast.vi"("error in (no error)"=w294, "Brake / Coast Mode"=w309, "CAN Jaguar Ref"=w295) -> ("error out"=w304:errorcluster, "CAN Jaguar Ref Out"=w303:T14)  [unwired: 7 in]
          n111 = call <vilib>:"WPI_CANJaguar_SetVoltageRampRate.vi"("error in (no error)"=w304, "VoltageRampRate (V/s)"=w300, "CAN Jaguar Ref"=w303) -> ("error out"=w286:errorcluster, "CAN Jaguar Ref Out"=w287:T14)  [unwired: 7 in]
          n112 = call <vilib>:"WPI_MotorControlRefNum Registry Set.vi"("error in (no error)"=w286, "refnum name"="Shooter Motor 2", "MotorControlDevRef"=w287) -> ("error out"=w281:errorcluster)  [unwired: 7 in, 1 out]
          n113 = call-poly <vilib>:"WPI_MotorControlOpen.vi"("Invert"=w279, "error in (no error)"=w281, "Device Number"=w314, "Control Mode"=w310) -> ("error out"=w292:errorcluster, "MotorControlDeviceRef"=w293:T14)  [unwired: 6 in]
          n114 = call <vilib>:"WPI_CANJaguar_ConfigBrakeCoast.vi"("error in (no error)"=w292, "Brake / Coast Mode"=w309, "CAN Jaguar Ref"=w293) -> ("error out"=w305:errorcluster, "CAN Jaguar Ref Out"=w306:T14)  [unwired: 7 in]
          n115 = call <vilib>:"WPI_CANJaguar_SetVoltageRampRate.vi"("error in (no error)"=w305, "VoltageRampRate (V/s)"=w300, "CAN Jaguar Ref"=w306) -> ("error out"=w284:errorcluster, "CAN Jaguar Ref Out"=w285:T14)  [unwired: 7 in]
          n116 = call <vilib>:"WPI_MotorControlRefNum Registry Set.vi"("error in (no error)"=w284, "refnum name"="Shooter Motor 1", "MotorControlDevRef"=w285) -> ("error out"=w277:errorcluster)  [unwired: 7 in, 1 out]
        }
        frame Disabled {
          w318 = TRUE  # Invert Motor Direction
          w332 = FPGA_TypedefDigitalModule."Digital Module 1"  # Digital Module
          # "This mode is disabled, and I hope we don't have to use it.\n\nNot much to comment here.  This is how the PWMs are opened on the Jaguars."
          # "PWM"
          n117 = call-poly <vilib>:"WPI_MotorControlOpen.vi"("Invert"=w318, "error in (no error)"=w323, "PWM Channel"=FPGA_DIOPWMChannel."PWM 8", "Digital Module (Module 1)"=w332) -> ("error out"=w327:errorcluster, "MotorControlDeviceRef"=w326:T14)  [unwired: 6 in]
          n118 = call <vilib>:"WPI_MotorControlRefNum Registry Set.vi"("error in (no error)"=w327, "refnum name"="Shooter Motor 4", "MotorControlDevRef"=w326) -> ("error out"=w322:errorcluster)  [unwired: 7 in, 1 out]
          n119 = call-poly <vilib>:"WPI_MotorControlOpen.vi"("Invert"=w318, "error in (no error)"=w322, "PWM Channel"=FPGA_DIOPWMChannel."PWM 7", "Digital Module (Module 1)"=w332) -> ("error out"=w329:errorcluster, "MotorControlDeviceRef"=w328:T14)  [unwired: 6 in]
          n120 = call <vilib>:"WPI_MotorControlRefNum Registry Set.vi"("error in (no error)"=w329, "refnum name"="Shooter Motor 3", "MotorControlDevRef"=w328) -> ("error out"=w321:errorcluster)  [unwired: 7 in, 1 out]
          n121 = call-poly <vilib>:"WPI_MotorControlOpen.vi"("Invert"=w318, "error in (no error)"=w321, "PWM Channel"=FPGA_DIOPWMChannel."PWM 6", "Digital Module (Module 1)"=w332) -> ("error out"=w325:errorcluster, "MotorControlDeviceRef"=w324:T14)  [unwired: 6 in]
          n122 = call <vilib>:"WPI_MotorControlRefNum Registry Set.vi"("error in (no error)"=w325, "refnum name"="Shooter Motor 2", "MotorControlDevRef"=w324) -> ("error out"=w320:errorcluster)  [unwired: 7 in, 1 out]
          n123 = call-poly <vilib>:"WPI_MotorControlOpen.vi"("Invert"=w318, "error in (no error)"=w320, "PWM Channel"=FPGA_DIOPWMChannel."PWM 5", "Digital Module (Module 1)"=w332) -> ("error out"=w331:errorcluster, "MotorControlDeviceRef"=w330:T14)  [unwired: 6 in]
          n124 = call <vilib>:"WPI_MotorControlRefNum Registry Set.vi"("error in (no error)"=w331, "refnum name"="Shooter Motor 1", "MotorControlDevRef"=w330) -> ("error out"=w319:errorcluster)  [unwired: 7 in, 1 out]
        }
      }
    }
  }
  n125 = disable-structure shown="Disabled" {
    frame Disabled {
      (unwired) string[][] [["Analog Port", "Description"], ["1", "Gyro"], ["2", ""], ["3", ""], ["4", ""], ["5", ""], ["6", ""], ["7", ""], ["8", "Battery (Internal)"]]  # Analog Module 1
      (unwired) string[][] [["I/O Port", "Description"], ["1", "Encoder A"], ["2", "Encoder B"], ["3", "Pressure Switch"], ["4", "Autonomous 1"], ["5", "Autonomous 2"], ["6", ""], ["7", ""], ["8", ""], ["9", ""], ["10", ""], ["11", ""], ["12", ""], ["13", ""], ["14", ""], ["15", ""], ["16", ""]]  # Digital Module 1 I/O
      (unwired) string[][] [["Relay Port", "Description"], ["1", "Compressor"], ["2", ""], ["3", ""], ["4", " "], ["5", ""], ["6", ""], ["7", ""], ["8", ""]]  # Digital Module 1 Relays
      (unwired) string[][] [["Solenoid Port", "Description"], ["1", "Arm FW"], ["2", "Arm BW"], ["3", "Shifter FW"], ["4", "Shifter BW"], ["5", ""], ["6", ""], ["7", ""], ["8", ""]]  # Solenoid Module 2
      (unwired) string[][] [["Solenoid Port", "Description"], ["1", "Shooter 2 FW"], ["2", "Shooter 2 BW"], ["3", "Ball Grabber FW"], ["4", "Ball Grabber BW"], ["5", "Shooter 1 FW"], ["6", "Shooter 1 BW"], ["7", "Horn FW"], ["8", "Horn BW"]]  # Solenoid Module 1
      (unwired) string[][] [["PWM Port", "Description"], ["1", "Left Drive 1"], ["2", "Left Drive 2"], ["3", "Right Drive 1"], ["4", "Right Drive 2"], ["5", "(Disabled) Shooter 1"], ["6", "(Disabled) Shooter 2"], ["7", "(Disabled) Shooter 3"], ["8", "(Disabled) Shooter 4"]]  # Digital Module 1 PWM
      # "This code has no functionality.  It serves as a reference if something gets disconnected."
      # "Inputs and Outputs for the 2012 Robot"
    }
    frame Enabled {
    }
  }
  n126 = Merge Errors(w2, w3, w10, w9, w8, w7, w6, w1) -> (w4:errorcluster)
  n127 = disable-structure shown="Enabled" {
    disable-tunnel: [w342 w345] -> w5
    disable-tunnel: w4 -> [w341 w345]
    frame Disabled {
      # "Timer, if needed..."
      n128 = flat-sequence {
        tunnel: [w344] -> w342
        tunnel: w341 -> [w344]
        frame #0 {
          n129 = Wait (ms)(milliseconds to wait=u32 5000) -> ()  [unwired: 1 out]
        }
      }
    }
    frame Enabled {
      # "No timer needed."
    }
  }
  "error out" <- w5
